vi "I2C_Query.vi"(0 "System no.":i32=1 min=1 max=4 step=1, 5 "error in":errorcluster) -> (14 "I²C status message":string, 19 "error out":errorcluster)   [LabVIEW 2020]
doc: "Returns the status message of the I²C bus.\n\nE-816: Status message consists of status bit and channel ID. This command cannot be issued to a slave."
panel:
  # "Returns the status message of the I²C bus."
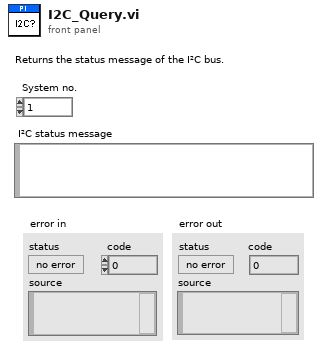
[diagram p1: front panel]
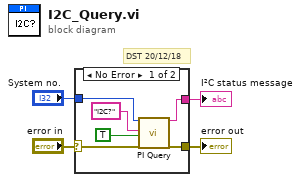
[diagram p0: block diagram]
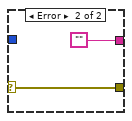
[diagram p2: hidden frame]
diagram:
  # "DST 20/12/18"
  n1 = case shown="No Error" "error in" {
    selector: "error in" -> [w7 w12]
    tunnel: [w6 "" ("String read")] -> w4
    tunnel: [w5 w12] -> w3
    tunnel: "System no." -> [w8 _]
    frame No Error {
      n2 = call "PI Query.vi"("System no."=w8, "String to send"="I2C?" ("String to Send"), "Attach termination char.?"=TRUE ("Attach Linefeed?"), "error in"=w7) -> ("String read"=w6:string, "error out"=w5:errorcluster)  [unwired: 3 in, 11 out]
    }
    frame Error {
    }
  }
  "I²C status message" <- w4
  "error out" <- w3
